vi "Macro Add.vi"(8 "error in (no error)":errorcluster, 11 "Git in":refnum<class "Git.lvclass">) -> (0 "error out":errorcluster, 3 "Git out":refnum<class "Git.lvclass">)   [LabVIEW 2019, in "Git.lvclass"]
uses:
  Git.lvclass
  Git.lvclass/Git.ctl
  <vilib>/Hampel Software Engineering/Git API/Git API/GIT-api.lvclass
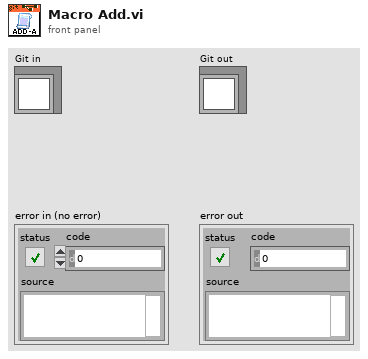
[diagram p1: front panel]
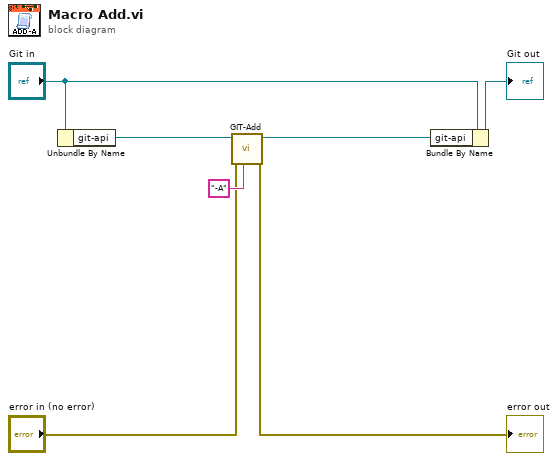
[diagram p0: block diagram]
diagram:
  n1 = Unbundle By Name("Git in") -> ("git-api"=w4:refnum<class "GIT-api.lvclass">)
  n2 = call <vilib>:"GIT-Add.vi"("param"="-A", "error in"="error in (no error)", "git-api in"=w4) -> ("error out"=→"error out":errorcluster, "git-api out"=w3:refnum<class "GIT-api.lvclass">)  [unwired: 6 in, 1 out]
  n3 = Bundle By Name(cluster="Git in", "git-api"=w3) -> (→"Git out":refnum<class "Git.lvclass">)
